vi "ICNC Move Speed Rel Local Buf.vi"(0 "Speed":u32, 1 "MoveA":i32, 2 "BufferRequired":u32, 5 "MoveX":i32, 7 "MoveY":i32, 9 "MoveZ":i32, 11 "error in (no error)":errorcluster caption="entrée d'erreur (pas d'erreur)", 12 "MoveB":i32) -> (4 "BufferRequired out":u32, 6 "function return":u32, 15 "error out":errorcluster caption="sortie d'erreur")   [LabVIEW 2012, in "ICNC2.lvlib"]
doc: "DWORD ICNC_MoveSpeedRelLocalBuf (DWORD Speed,\n INT MoveX,\n INT MoveY,\n INT MoveZ,\n INT MoveA,\n INT MoveB,\n DWORD *BufferRequired=NULL);"
uses:
  <userlib>/ICNC/ICNC2.lvlib
  <userlib>/ICNC/ICNC2.dll
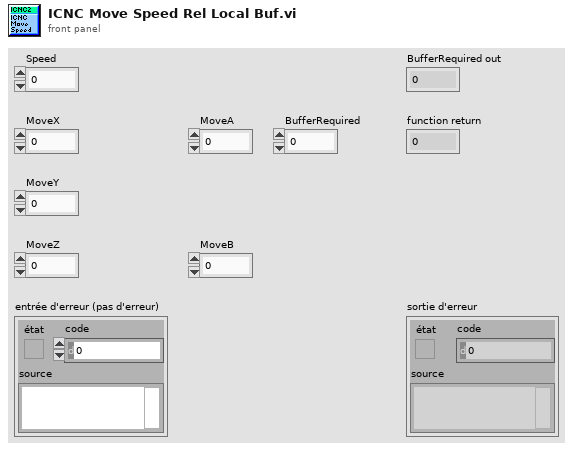
[diagram p1: front panel]
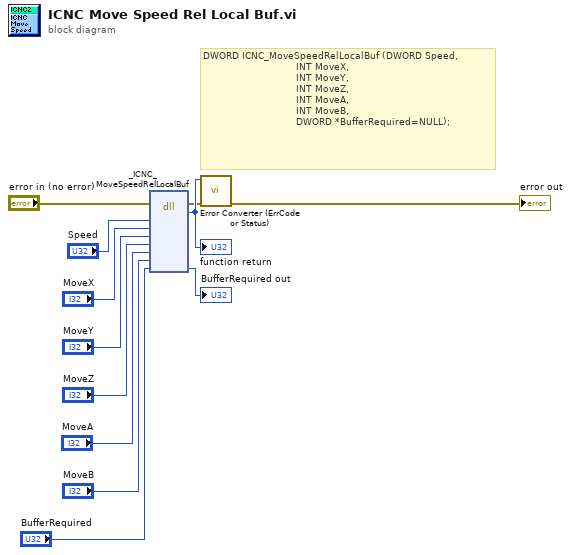
[diagram p0: block diagram]
diagram:
  # "DWORD ICNC_MoveSpeedRelLocalBuf (DWORD Speed,\n                               INT MoveX,\n                               INT MoveY,\n                               INT MoveZ,\n                               INT MoveA,\n                               INT MoveB,\n                               DWORD *BufferRequired=NULL);"
  n1 = dll-call lib="C:/Program Files (x86)/National Instruments/LabVIEW 2012/user.lib/ICNC/ICNC2.*" fn="_ICNC_MoveSpeedRelLocalBuf"(error in="error in (no error)", "Speed"="Speed", "MoveX"="MoveX", "MoveY"="MoveY", "MoveZ"="MoveZ", "MoveA"="MoveA", "MoveB"="MoveB", "BufferRequired"="BufferRequired") -> (error out=w2:errorcluster, w12:u32, "BufferRequired"=→"BufferRequired out":u32)  [unwired: 8 in, 1 out]
  "function return" <- w12
  n2 = call <userlib>:"Error Converter (ErrCode or Status).vi"("error in (no error)"=w2, "error code"=w12) -> ("error out"=→"error out":errorcluster)  [unwired: 9 in]
